vi "Get Performance.vi"(11 "Framework in":refnum<class "Framework.lvclass">) -> (2 "Performance":refnum<class "Performance.lvclass">, 3 "Framework out":refnum<class "Framework.lvclass">)   [LabVIEW 2020, in "DSF Core.lvlib" / "Framework.lvclass"]
uses:
  Framework.lvclass
  Performance/Performance.lvclass
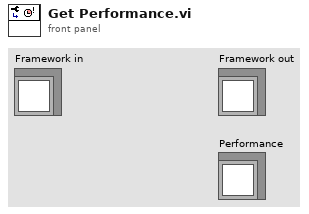
[diagram p1: front panel]
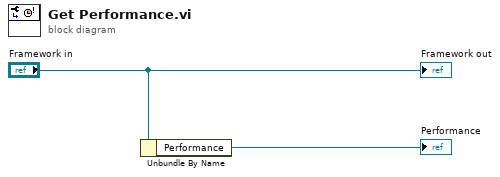
[diagram p0: block diagram]
diagram:
  n1 = Unbundle By Name("Framework in") -> ("Performance"=→"Performance":refnum<class "Performance.lvclass">)
  "Framework out" <- "Framework in"
